vi "Create Object (drawable).vi"(8 "error in (no error)":errorcluster, 10 "Geometry":refnum<vi>, 11 "Name":string) -> (0 "error out":errorcluster, 3 "Scene:New Object":refnum<vi>)   [LabVIEW 2020, in "NI_3D Picture Control.lvlib"]
doc: "Creates a new 3D object to display in the 3D scene."
uses:
  <vilib>/picture/3D Picture Control/NI_3D Picture Control.lvlib
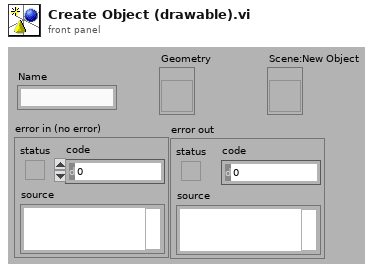
[diagram p1: front panel]
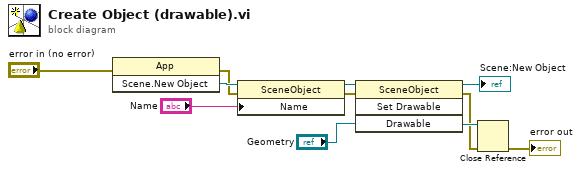
[diagram p0: block diagram]
diagram:
  n1 = invoke class="App" method="Scene.New Object"(error in="error in (no error)") -> (error out=w9:errorcluster, "Scene.New Object"=w10:refnum<vi>)  [unwired: 2 in, 1 out]
  n2 = property class="SceneObject"(reference=w10, error in=w9, "Name"="Name") -> (reference out=w7:refnum<vi>, error out=w6:errorcluster)
  n3 = invoke class="SceneObject" method="Set Drawable"(reference=w7, error in=w6, "Drawable"="Geometry") -> (reference out=→"Scene:New Object":refnum<vi>, error out=w2:errorcluster, "Drawable"=w3:refnum<vi>)  [unwired: 1 in, 1 out]
  n4 = Close Reference(reference=w3, error in (no error)=w2) -> (error out=→"error out":errorcluster)
